vi "SPI_Write.vi"(0 "Handle":u32, 1 "WriteStartCondition":T4 {"Chip Select Pin" items=["Chip Select (ADBUS3)", "GPIOL1 (ADBUS4)", "GPIOL2 (ADBUS5)", "GPIOL3 (ADBUS6)", "GPIOL4 (ADBUS7)"]}, 2 "Control and Data Bits":T2={"ClockOutDataBitsMSBFirst"=FALSE, "ClockOutDataBitsPosEdge"=FALSE, "NumControlBitsToWrite"=2, "WriteControlBuffer"=[], "NumControlBytesToWrite"=1, "WriteDataBits"=FALSE, "NumDataBitsToWrite"=2, "WriteDataBuffer"=[], "NumDataBytesToWrite"=1} {"NumDataBytesToWrite" min=1 max=65535; "WriteDataBuffer" format="%x"; "NumDataBitsToWrite" min=2 max=524280; "NumControlBytesToWrite" min=1 max=255; "WriteControlBuffer" format="%x"; "NumControlBitsToWrite" min=2 max=2040}, 3 "WaitDataWriteComplete":T1 {"WaitDataWritePin" items=["Data In (ADBUS2)", "GPIOH1 (ACBUS0)", "GPIOH2 (ACBUS1)", "GPIOH3 (ACBUS2)", "GPIOH4 (ACBUS3)"]}, 4 "HighPinsWriteActiveStates":T3) -> (5 "FTC_Status":u32)   [LabVIEW 2010]
uses:
  WINNT/system32/FTCSPI.dll
panel:
  out "size(s)":i32
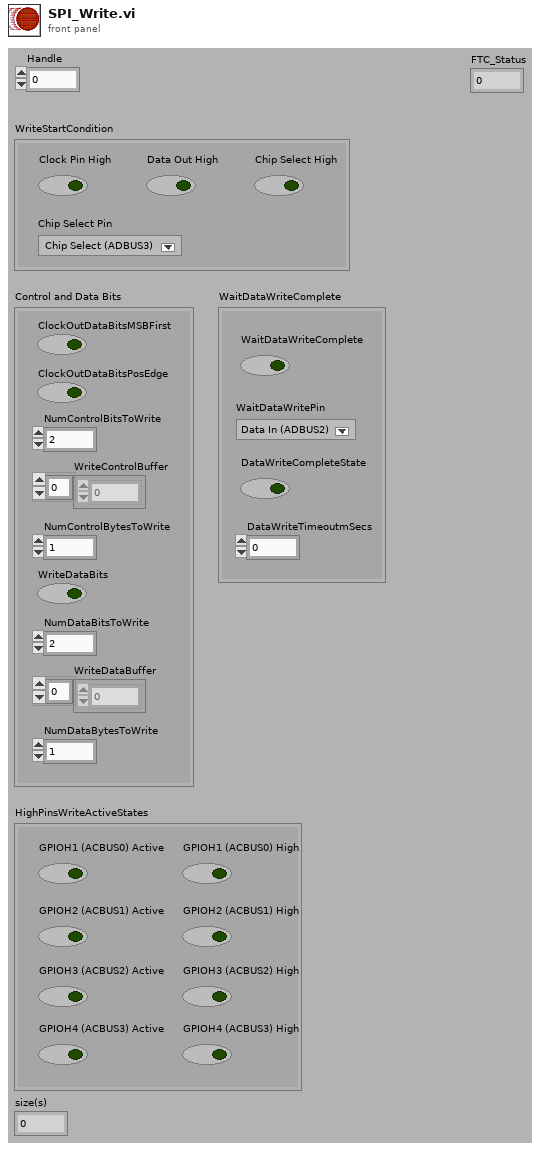
[diagram p1: front panel]
types:
  T1 = cluster{"WaitDataWriteComplete":bool, "WaitDataWritePin":u32, "DataWriteCompleteState":bool, "DataWriteTimeoutmSecs":u32}
  T2 = cluster{"ClockOutDataBitsMSBFirst":bool, "ClockOutDataBitsPosEdge":bool, "NumControlBitsToWrite":u32, "WriteControlBuffer":u8[], "NumControlBytesToWrite":u32, "WriteDataBits":bool, "NumDataBitsToWrite":u32, "WriteDataBuffer":u8[], "NumDataBytesToWrite":u32}
  T3 = cluster{"GPIOH1 (ACBUS0) Active":bool, "GPIOH1 (ACBUS0) High":bool, "GPIOH2 (ACBUS1) Active":bool, "GPIOH2 (ACBUS1) High":bool, "GPIOH3 (ACBUS2) Active":bool, "GPIOH3 (ACBUS2) High":bool, "GPIOH4 (ACBUS3) Active":bool, "GPIOH4 (ACBUS3) High":bool}
  T4 = cluster{"Clock Pin High":bool, "Data Out High":bool, "Chip Select High":bool, "Chip Select Pin":u32}
  T5 = cluster{u32, "WaitDataWritePin":u32, u32, "DataWriteTimeoutmSecs":u32}
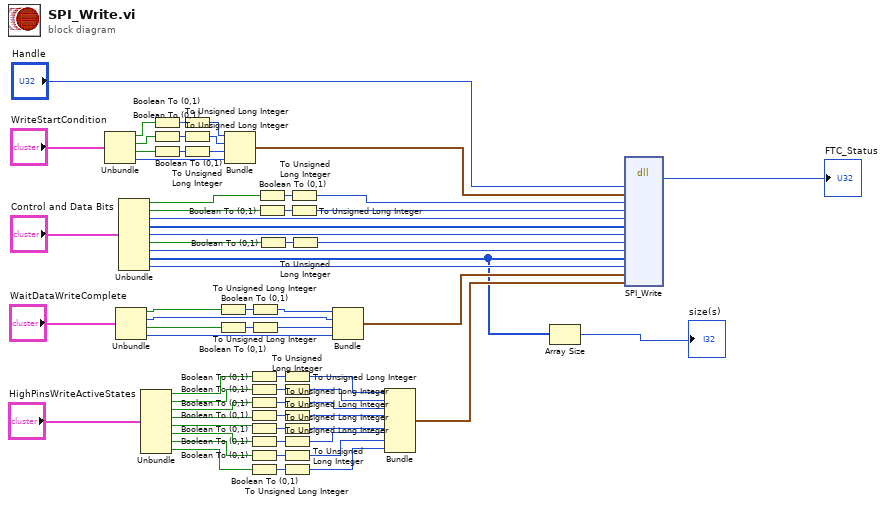
[diagram p0: block diagram]
diagram:
  n1 = Unbundle("WriteStartCondition") -> ("Clock Pin High"=w64:bool, "Data Out High"=w61:bool, "Chip Select High"=w60:bool, "Chip Select Pin"=w56:u32)
  n2 = Unbundle("WaitDataWriteComplete") -> ("WaitDataWriteComplete"=w9:bool, "WaitDataWritePin"=w6:u32, "DataWriteCompleteState"=w8:bool, "DataWriteTimeoutmSecs"=w4:u32)
  n3 = Unbundle("Control and Data Bits") -> ("ClockOutDataBitsMSBFirst"=w27:bool, "ClockOutDataBitsPosEdge"=w26:bool, "NumControlBitsToWrite"=w25:u32, "WriteControlBuffer"=w24:u8[], "NumControlBytesToWrite"=w23:u32, "WriteDataBits"=w15:bool, "NumDataBitsToWrite"=w14:u32, "WriteDataBuffer"=w2:u8[], "NumDataBytesToWrite"=w13:u32)
  n4 = Unbundle("HighPinsWriteActiveStates") -> ("GPIOH1 (ACBUS0) Active"=w45:bool, "GPIOH1 (ACBUS0) High"=w44:bool, "GPIOH2 (ACBUS1) Active"=w43:bool, "GPIOH2 (ACBUS1) High"=w42:bool, "GPIOH3 (ACBUS2) Active"=w41:bool, "GPIOH3 (ACBUS2) High"=w40:bool, "GPIOH4 (ACBUS3) Active"=w39:bool, "GPIOH4 (ACBUS3) High"=w38:bool)
  n5 = Boolean To (0,1)(Boolean=w64) -> (0, 1=w65:i16)
  n6 = Boolean To (0,1)(Boolean=w61) -> (0, 1=w63:i16)
  n7 = Boolean To (0,1)(Boolean=w60) -> (0, 1=w62:i16)
  n8 = To Unsigned Long Integer(number=w65) -> (unsigned 32bit integer=w59:u32)
  n9 = To Unsigned Long Integer(number=w63) -> (unsigned 32bit integer=w58:u32)
  n10 = To Unsigned Long Integer(number=w62) -> (unsigned 32bit integer=w57:u32)
  n11 = Boolean To (0,1)(Boolean=w9) -> (0, 1=w11:i16)
  n12 = Boolean To (0,1)(Boolean=w8) -> (0, 1=w10:i16)
  n13 = Bundle(w59, w58, w57, "Chip Select Pin"=w56) -> (w22:cluster{u32, u32, u32, "Chip Select Pin":u32})  [unwired: 1 in]
  n14 = Boolean To (0,1)(Boolean=w45) -> (0, 1=w52:i16)
  n15 = Boolean To (0,1)(Boolean=w44) -> (0, 1=w51:i16)
  n16 = Boolean To (0,1)(Boolean=w43) -> (0, 1=w50:i16)
  n17 = Boolean To (0,1)(Boolean=w42) -> (0, 1=w49:i16)
  n18 = Boolean To (0,1)(Boolean=w41) -> (0, 1=w48:i16)
  n19 = Boolean To (0,1)(Boolean=w40) -> (0, 1=w47:i16)
  n20 = Boolean To (0,1)(Boolean=w39) -> (0, 1=w46:i16)
  n21 = Boolean To (0,1)(Boolean=w38) -> (0, 1=w53:i16)
  n22 = To Unsigned Long Integer(number=w11) -> (unsigned 32bit integer=w7:u32)
  n23 = To Unsigned Long Integer(number=w10) -> (unsigned 32bit integer=w5:u32)
  n24 = Boolean To (0,1)(Boolean=w27) -> (0, 1=w55:i16)
  n25 = Boolean To (0,1)(Boolean=w26) -> (0, 1=w54:i16)
  n26 = Boolean To (0,1)(Boolean=w15) -> (0, 1=w17:i16)
  n27 = To Unsigned Long Integer(number=w52) -> (unsigned 32bit integer=w37:u32)
  n28 = To Unsigned Long Integer(number=w51) -> (unsigned 32bit integer=w36:u32)
  n29 = To Unsigned Long Integer(number=w50) -> (unsigned 32bit integer=w35:u32)
  n30 = To Unsigned Long Integer(number=w49) -> (unsigned 32bit integer=w34:u32)
  n31 = To Unsigned Long Integer(number=w48) -> (unsigned 32bit integer=w33:u32)
  n32 = To Unsigned Long Integer(number=w47) -> (unsigned 32bit integer=w32:u32)
  n33 = To Unsigned Long Integer(number=w46) -> (unsigned 32bit integer=w31:u32)
  n34 = To Unsigned Long Integer(number=w53) -> (unsigned 32bit integer=w30:u32)
  n35 = To Unsigned Long Integer(number=w55) -> (unsigned 32bit integer=w19:u32)
  n36 = To Unsigned Long Integer(number=w54) -> (unsigned 32bit integer=w20:u32)
  n37 = To Unsigned Long Integer(number=w17) -> (unsigned 32bit integer=w16:u32)
  n38 = Bundle(w7, "WaitDataWritePin"=w6, w5, "DataWriteTimeoutmSecs"=w4) -> (w3:T5)  [unwired: 1 in]
  n39 = Bundle(w37, w36, w35, w34, w33, w32, w31, w30) -> (w18:cluster{u32, u32, u32, u32, u32, u32, u32, u32})  [unwired: 1 in]
  n40 = Array Size(array=w2) -> (size(s)=→"size(s)":i32)
  n41 = dll-call lib="C:/Users/WINNT/system32/FTCSPI.dll" fn="SPI_Write"("Handle"="Handle", w22, "ClockOutControlBitsMSBFirst"=w19, "ClockOutControlBitsPosEdge"=w20, "NumControlBitsToWrite"=w25, "WriteControlBuffer"=w24, "NumControlBytesToWrite"=w23, "WriteDataBits"=w16, "NumDataBitsToWrite"=w14, "WriteDataBuffer"=w2, "NumDataBytesToWrite"=w13, w3, w18) -> ("FTC_Status"=→"FTC_Status":u32)  [unwired: 16 in, 2 out]
